vi "dfd_Set Bank Type Infos.vi"(6 "filter bank type":T1 items=["Uniform", "Non-Uniform"], 8 "error in (no error)":errorcluster, 9 "processing method":T2, 10 "subband filters":T4[](array[typedef]) {"mMRate_SumWl" min=1 max=32 step=1; "mMRate_InputIwl" min=1 max=32 step=1; "mMRate_GainWl" min=1 max=32 step=1; "mMRate_OutputWl" min=1 max=32 step=1; "mMRate_InputWl" min=1 max=32 step=1; "mMRate_CoefWl" min=1 max=32 step=1; "mMRate_Mode" items=["Default"=-1, "No Rate Change"=0, "Interpolation"=1, "Decimation"=2, "Interpolated"=3, "Rational"=4]}, 11 "bank in":T3={"mBank_Filters"=[], " mBank_#Bands"=2, "mBank_ProcMethod"=enum."General", "mBank_Coeffs"=[], "mBank_Gain"=1.0, "mBank_Type"=0} {"mBank_Type" items=["Uniform", "Non-Uniform"]; "mBank_Filters"."mMRate_SumWl" min=1 max=32 step=1; "mBank_Filters"."mMRate_InputIwl" min=1 max=32 step=1; "mBank_Filters"."mMRate_GainWl" min=1 max=32 step=1; "mBank_Filters"."mMRate_OutputWl" min=1 max=32 step=1; "mBank_Filters"."mMRate_InputWl" min=1 max=32 step=1; "mBank_Filters"."mMRate_CoefWl" min=1 max=32 step=1; "mBank_Filters"."mMRate_Mode" items=["Default"=-1, "No Rate Change"=0, "Interpolation"=1, "Decimation"=2, "Interpolated"=3, "Rational"=4]}) -> (0 "error out":errorcluster, 3 "bank out":T3={"mBank_Filters"=[], " mBank_#Bands"=2, "mBank_ProcMethod"=enum."General", "mBank_Coeffs"=[], "mBank_Gain"=1.0, "mBank_Type"=0} {"mBank_Type" items=["Uniform", "Non-Uniform"]; "mBank_Filters"."mMRate_SumWl" min=1 max=32 step=1; "mBank_Filters"."mMRate_InputIwl" min=1 max=32 step=1; "mBank_Filters"."mMRate_GainWl" min=1 max=32 step=1; "mBank_Filters"."mMRate_OutputWl" min=1 max=32 step=1; "mBank_Filters"."mMRate_InputWl" min=1 max=32 step=1; "mBank_Filters"."mMRate_CoefWl" min=1 max=32 step=1; "mBank_Filters"."mMRate_Mode" items=["Default"=-1, "No Rate Change"=0, "Interpolation"=1, "Decimation"=2, "Interpolated"=3, "Rational"=4]})   [LabVIEW 2017, in "NI_DigFilter_FilterBank.lvlib"]
uses:
  <vilib>/addons/Digital Filter Design/NI_DigFilter_FilterBank.lvlib
  <vilib>/addons/Digital Filter Design/_Objects.llb/DFD Multirate Filter Obj.ctl
  <vilib>/addons/Digital Filter Design/_Objects.llb/DFD Multirate Mode.ctl
  <vilib>/addons/Digital Filter Design/_Objects.llb/DFD Coef Norm Type.ctl
  <vilib>/addons/Digital Filter Design/_Objects.llb/DFD Round-off Mode.ctl
  <vilib>/addons/Digital Filter Design/_Objects.llb/DFD FXP MRate Multiply Mode.ctl
  <vilib>/addons/Digital Filter Design/FilterBank.llb/Object/DFD Bank Obj.ctl
  <vilib>/addons/Digital Filter Design/FilterBank.llb/Object/DFD Filter Bank Processing Method.ctl
  <vilib>/addons/Digital Filter Design/FilterBank.llb/Object/DFD Filter Bank Type.ctl
  <vilib>/addons/Digital Filter Design/_Misc.llb/dfd_Error Handlers (Single).vi
  <vilib>/addons/Digital Filter Design/NI_DigFilterLicensed.lvlib
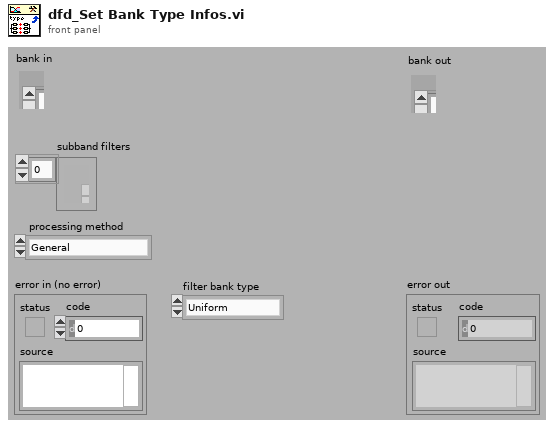
[diagram p1: front panel]
types:
  T1 = typedef "NI_DigFilter_FilterBank.lvlib/DFD Filter Bank Type.ctl" = u16
  T2 = typedef "NI_DigFilter_FilterBank.lvlib/DFD Filter Bank Processing Method.ctl" = enum16{"General", "2-Band QMF Lattice", "Cosine-Modulated"}
  T3 = typedef "NI_DigFilter_FilterBank.lvlib/DFD Bank Obj.ctl" = cluster{"mBank_Filters":T4[], " mBank_#Bands":i32, "mBank_ProcMethod":T2, "mBank_Coeffs":dbl[], "mBank_Gain":dbl, "mBank_Type":T1}
  T4 = typedef "NI_DigFilterLicensed.lvlib/DFD Multirate Filter Obj.ctl" = cluster{"mMRate_Structure":enum16{"CIC", "FIR", "IIR", "Lattice"}, "mMRate_Mode":T5, "mMRate_Factor":i32, "mMRate_FIRParams":cluster{"mMRate_FIR_H":dbl[], "mMRate_FIR_IsNyquist?":bool, "mMRate_FIR_IsSymmetric?":bool}, "mMRate_CICParams":cluster{"mMRate_CIC_#Stage":i32, "mMRate_CIC_Lag":i32, "mMRate_CIC_Type":enum16{"Lowpass", "Highpass"}}, "mMRate_Order":i32, "mMRate_Version":string, "mMRate_Comments":string, "mMRate_RationalFactor":cluster{"mMRate_L":i32, "mMRate_M":i32}, "mMRate_Fs":dbl, "mMRate_Quantized?":bool, "mMRate_QFilterGain":dbl, "mMRate_CoefWl":i16, "mMRate_Scaling":cluster{"mMRate_ScaleByPowerOf2?":bool, "mMRate_ScaleType":T6}, "mMRate_InputWl":i16, "mMRate_OutputWl":i16, "mMRate_OutputMode":T7, "mMRate_MultMode":T8, "mMRate_BitPruning":bool, "mMRate_GainWl":i16, "mMRate_OutputFwl":i16, "mMRate_SumIwl":i16, "mMRate_InputIwl ":i16, "mMRate_SumWl":i16, "mMRate_CoefIwl":i16}
  T5 = typedef "NI_DigFilterLicensed.lvlib/DFD Multirate Mode.ctl" = i16
  T6 = typedef "NI_DigFilterLicensed.lvlib/DFD Coef Norm Type.ctl" = enum16{"No Norm", "Time Domain 1-Norm", "Time Domain 2-Norm", "Time Domain Inf-Norm"}
  T7 = typedef "NI_DigFilterLicensed.lvlib/DFD Round-off Mode.ctl" = enum16{"Nearest", "Truncation"}
  T8 = typedef "NI_DigFilterLicensed.lvlib/DFD FXP MRate Multiply Mode.ctl" = enum16{"Truncated", "Full"}
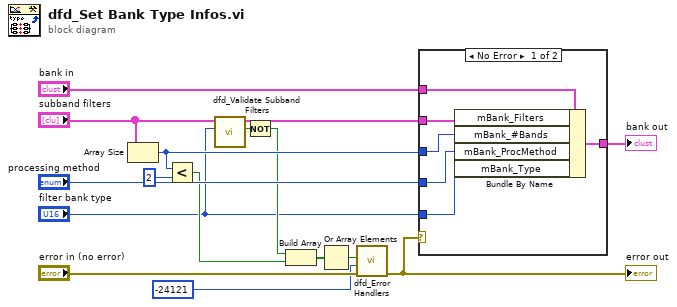
[diagram p0: block diagram]
diagram:
  n1 = Array Size(array="subband filters") -> (size(s)=w9:i32)
  n2 = Less?(x=w9, y=2) -> (x < y?=w4:bool)
  n3 = call <vilib>:"dfd_Validate Subband Filters.vi"("filter bank structure"="filter bank type", "subband filters in"="subband filters") -> ("is Valid?"=w10:bool, "subband filters out"=w11:T4[])  [unwired: 6 in, 2 out]
  n4 = Not(x=w10) -> (.not. x?=w5:bool)
  n5 = Build Array(w5, w4) -> (w8:bool[])
  n6 = Or Array Elements(Boolean array=w8) -> (logical OR=w3:bool)
  n7 = call-poly <vilib>:"dfd_Error Handlers.vi"("error in (no error)"="error in (no error)", "error code"=-24121 ("ERR_INVALID_FILTERBANK_OBJ"), "condition failed?"=w3) -> ("error out"=w6:errorcluster)  [unwired: 8 in]
  "error out" <- w6
  n8 = case shown="No Error" w6 {
    tunnel: "processing method" -> [w22 _]
    tunnel: "bank in" -> [w21 w23]
    tunnel: w9 -> [w20 _]
    tunnel: w11 -> [w19 _]
    tunnel: [w18 w23] -> w14
    tunnel: "filter bank type" -> [w17 _]
    frame No Error {
      n9 = Bundle By Name(cluster=w21, "mBank_Filters"=w19, "mBank_#Bands"=w20, "mBank_ProcMethod"=w22, "mBank_Type"=w17) -> (w18:T3)
    }
    frame Error {
    }
  }
  "bank out" <- w14
